vi "Operation Status Query.vi"(0 "VISA resource name":refnum<visa-resource-name>, 11 "error in (no error)":errorcluster) -> (4 "VISA resource name out":refnum<visa-resource-name>, 6 "Operation Status":T1, 15 "error out":errorcluster)   [LabVIEW 2020, in "NH Research Regenerative Test Series.lvlib"]
doc: "Returns the integer data explaining the operation status monitored in the instrument.\n\nThe Operation Register consists of the following 16 bits:\n\nBit 0: Ready\nBit 1: Reserved\nBit 2: Reserved \nBit 3: Sweeping\nBit 4: Measuring\nBit 5: Waiting for Trigger \nBit 6: Trigger Detected\nBit 7: Reserved\nBit 8: Reserved\nBit 9: Active Mode Bit 0\nBit 10: Active Mode Bit 1\nBit 11: Active Mode Bit 2\nBit 12: Reserved\nBit 13: Reserved\nBit 14: Reserved\nBit 15: Reserved"
uses:
  NH Research Regenerative Test Series.lvlib
panel:
  # "Bit 0:  Ready\nBit 1:  Reserved\nBit 2:  Reserved\t\nBit 3:  Sweeping\nBit 4:\t\tMeasuring\nBit 5:  Waiting for Trigger\t\nBit 6:  Trigger Detected\nBit 7:  Reserved\nBit 8:  Reserved\nBit 9:  Active Mode Bit 0\nBit 10:  Active Mode Bit 1\nBit 11:  Active Mode Bit 2\nBit 12:  Reserved\nBit 13:  Reserved\nBit 14:  Reserved\nBit 15:  Reserved"
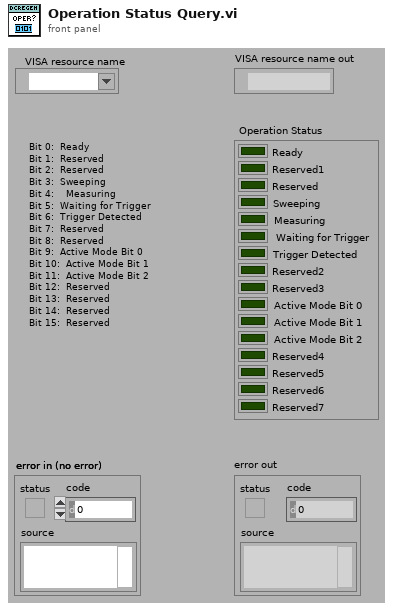
[diagram p1: front panel]
types:
  T1 = cluster{"Ready":bool, "Reserved1":bool, "Reserved":bool, "Sweeping":bool, "Measuring":bool, "Waiting for Trigger\t":bool, "Trigger Detected":bool, "Reserved2":bool, "Reserved3":bool, "Active Mode Bit 0":bool, "Active Mode Bit 1":bool, "Active Mode Bit 2":bool, "Reserved4":bool, "Reserved5":bool, "Reserved6":bool, "Reserved7":bool}
  T2 = cluster{"Operation Complete":bool, "Not Used":bool, "Query Error":bool, "Device Error":bool, "Message Available":bool, "Command Error":bool, "Not Used":bool, "Power On":bool, "Operation Complete 2":bool, "Not Used 2":bool, "Query Error 2":bool, "Device Error 2":bool, "Message Available 2":bool, "Command Error 2":bool, "Not Used 3":bool, "Power On 2":bool}
  T3 = cluster{"Boolean array[0]":bool, "Boolean array[1]":bool, "Boolean array[2]":bool, "Boolean array[3]":bool, "Boolean array[4]":bool, "Boolean array[5]":bool, "Boolean array[6]":bool, "Boolean array[7]":bool, "Boolean array[8]":bool, "Boolean array[9]":bool, "Boolean array[10]":bool, "Boolean array[11]":bool, "Boolean array[12]":bool, "Boolean array[13]":bool, "Boolean array[14]":bool, "Boolean array[15]":bool}
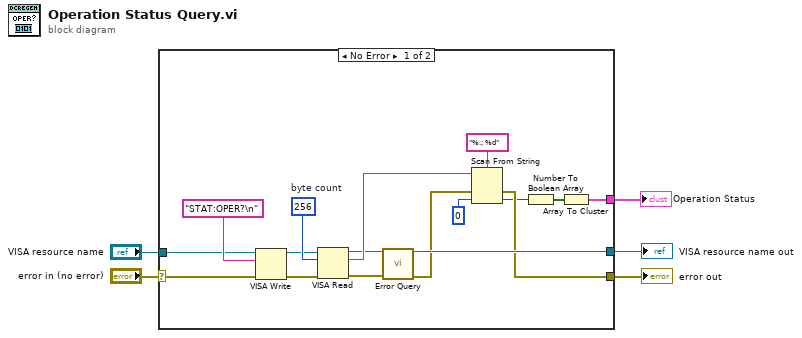
[diagram p0: block diagram]
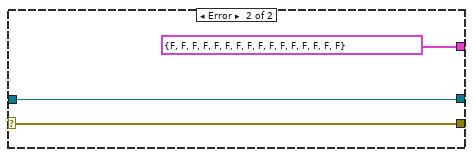
[diagram p2: hidden frame]
diagram:
  n1 = case shown="No Error" "error in (no error)" {
    selector: "error in (no error)" -> [w15 w25]
    tunnel: [w10 w25] -> w5
    tunnel: [w14 w24] -> w4
    tunnel: "VISA resource name" -> [w16 w24]
    tunnel: [w7 T2 {"Operation Complete"=FALSE, "Not Used"=FALSE, "Query Error"=FALSE, "Device Error"=FALSE, "Message Available"=FALSE, "Command Error"=FALSE, "Not Used"=FALSE, "Power On"=FALSE, "Operation Complete 2"=FALSE, "Not Used 2"=FALSE, "Query Error 2"=FALSE, "Device Error 2"=FALSE, "Message Available 2"=FALSE, "Command Error 2"=FALSE, "Not Used 3"=FALSE, "Power On 2"=FALSE} ("Operation Status")] -> w1
    frame No Error {
      w21 = u32 256  # byte count
      n2 = VISA Write(VISA resource name=w16, write buffer="STAT:OPER?\n" ("Command to Send (empty)"), error in (no error)=w15) -> (VISA resource name out=w19:refnum<visa-resource-name>, error out=w18:errorcluster)  [unwired: 1 out]
      n3 = VISA Read(VISA resource name=w19, byte count=w21, error in (no error)=w18) -> (VISA resource name out=w13:refnum<visa-resource-name>, read buffer=w20:string, error out=w12:errorcluster)  [unwired: 1 out]
      n4 = call "Error Query.vi"("VISA resource name"=w13, "error in (no error)"=w12) -> ("VISA resource name out"=w14:refnum<visa-resource-name>, "error out"=w11:errorcluster)  [unwired: 10 in, 2 out]
      n5 = Scan From String(format string="%.; %d" ("Format String"), input string=w20, error in=w11, default 1=u16 0 ("default value 1")) -> (error out=w10:errorcluster, output 1=w6:u16)  [unwired: 1 in, 2 out]
      n6 = Number To Boolean Array(number=w6) -> (Boolean array=w9:bool[])
      n7 = Array To Cluster(array=w9) -> (cluster=w7:T3)
    }
    frame Error {
    }
  }
  "error out" <- w5
  "VISA resource name out" <- w4
  "Operation Status" <- w1
